vi "Wait SubVI.vi"(10 "time (ms)":string, 11 "waiting":bool) -> (2 "timer value":u32, 3 "keep waiting":bool)   [LabVIEW 2019, in "SMO.Transport.lvclass"]
uses:
  SMO.Transport.lvclass
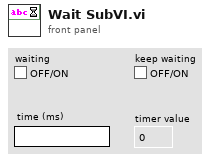
[diagram p1: front panel]
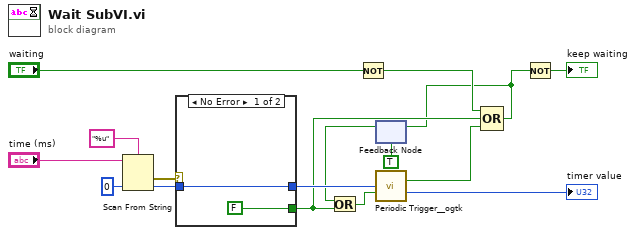
[diagram p0: block diagram]
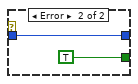
[diagram p2: hidden frame]
diagram:
  n1 = Scan From String(format string="%u", input string="time (ms)", default 1=u32 0 ("default value 1")) -> (error out=w4:errorcluster, output 1=w2:u32)  [unwired: 2 in, 2 out]
  n2 = case shown="No Error" w4 {
    tunnel: [w17 w19] -> w15
    tunnel: [FALSE ("y") TRUE ("y")] -> w10
    tunnel: w2 -> [w17 w19]
    frame No Error {
    }
    frame Error {
    }
  }
  n3 = Not(x="waiting") -> (.not. x?=w8:bool)
  n4 = feedback #1(TRUE ("Triggered")) -> (w14:bool)
  n5 = Or(x=w14, y=w10) -> (x .or. y?=w13:bool)
  n6 = call <userlib>:"Periodic Trigger__ogtk.vi"("time (ms)"=w15, "reset"=w13) -> ("Triggered"=w11:bool, "timer value"=→"timer value":u32)  [unwired: 11 in, 1 out]
  n7 = Compound Arithmetic op=OR(w8, w10, w11) -> (w7:bool)
  n8 = feedback-in #1(w7) -> ()
  n9 = Not(x=w7) -> (.not. x?=→"keep waiting":bool)
